vi "DAQ Data Variable.vi"() -> ()   [LabVIEW 2012]
panel:
  out "DAQ Variable":dbl[](array[numeric])
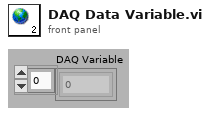
[diagram p1: front panel]
diagram:
